vi "Generic command handler.vi"(8 "error in (no error)":errorcluster, 10 "Message in":refnum<class "GenericMessage.lvclass">, 11 "Tomo in":refnum<class "Tomo.lvclass">) -> (0 "error out":errorcluster, 2 "value":string, 3 "Tomo out":refnum<class "Tomo.lvclass">)   [LabVIEW 2012, in "Tomo.lvclass"]
doc: "The generic_command_handler processes the command 'generic'. Commands which are not part of the predefined list of commands fall under the 'generic' command for special activity."
uses:
  Tomo.lvclass
  <vilib>/Distrio/Murmex/GenericMessage/GenericMessage.lvclass
  <vilib>/Distrio/Murmex/Murmex/Murmex.lvclass
  Tomo.lvclass/Tomo.ctl
  <vilib>/Distrio/Murmex/StartMessage/StartMessage.lvclass
  Current activity.ctl
  file type.ctl
  notice type.ctl
  <vilib>/Distrio/Murmex/StopMessage/StopMessage.lvclass
  <vilib>/Distrio/Murmex/Message/Add or replace parameter.vi
  <vilib>/Distrio/Murmex/Message/Message.lvclass
  <vilib>/vision/NI_Vision_Development_Module.lvlib
panel:
  out "Image 2":T1(plugin-control)
  out "Image":T1(plugin-control)
  # "This method is called when the GENERIC\ntrigger is sent. \n\nOverride this method when your component needs to\nrespond to this trigger. \n\nCall parent for proper implementation"
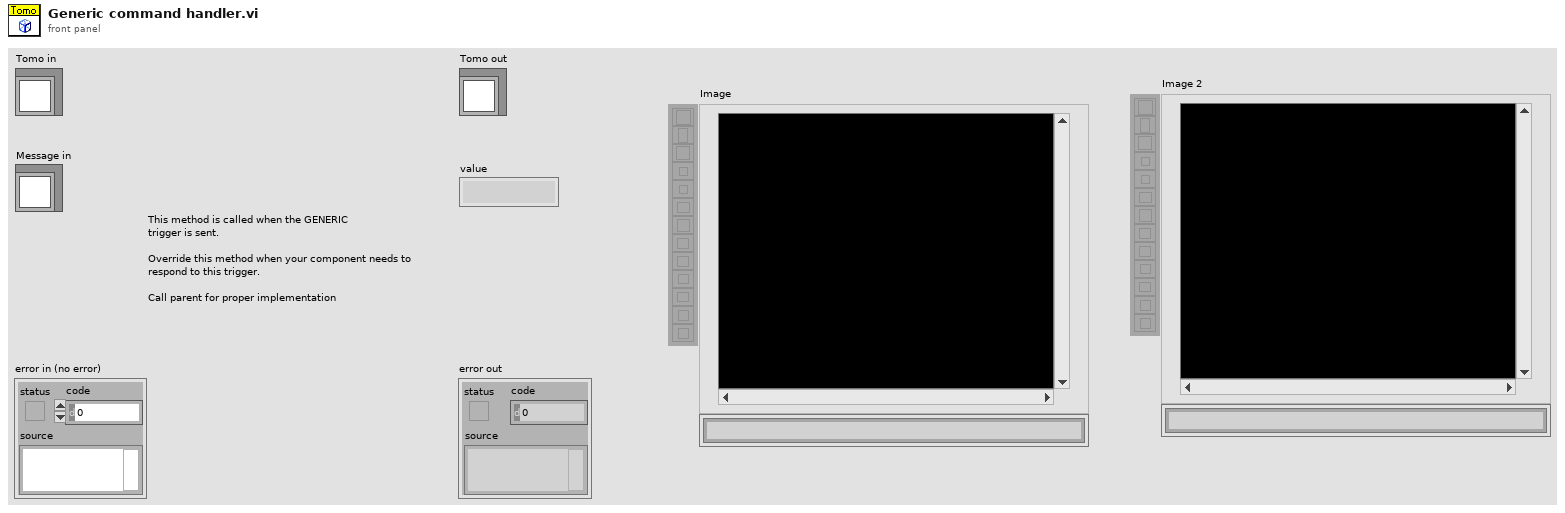
[diagram p1: front panel]
types:
  T1 = typedef "IMAQ Image.ctl" = refnum<image>
  T2 = typedef "Tomo.lvclass/Current activity.ctl" = enum16{"Idle", "Inter-stack motion", "Pre-tomo calculation", "Stack acquisition", "Stack preparation", "Pre-tomo stack acq", "Pre-tomo inter-stack"}
  T3 = typedef "Tomo.lvclass/file type.ctl" = enum16{"Volume map", "Completed stacks"}
  T4 = typedef "Tomo.lvclass/notice type.ctl" = enum16{"Tomography stopped", "Tomography error", "Tomography finished", "Timing issue", "Critical timing issue"}
  T5 = typedef "Tomo.lvclass/volume map.ctl" = enum16{"Cubic volume", "Custom volume", "Self-generate volume", "Time- tomography"}
  T6 = cluster{"Mean Value":sgl, "Standard Variation":sgl, "Minimal Value":sgl, "Maximal Value":sgl, "Area (calibrated)":sgl, "Area (pixels)":u32, "%":sgl, "Calibration Valid":bool}
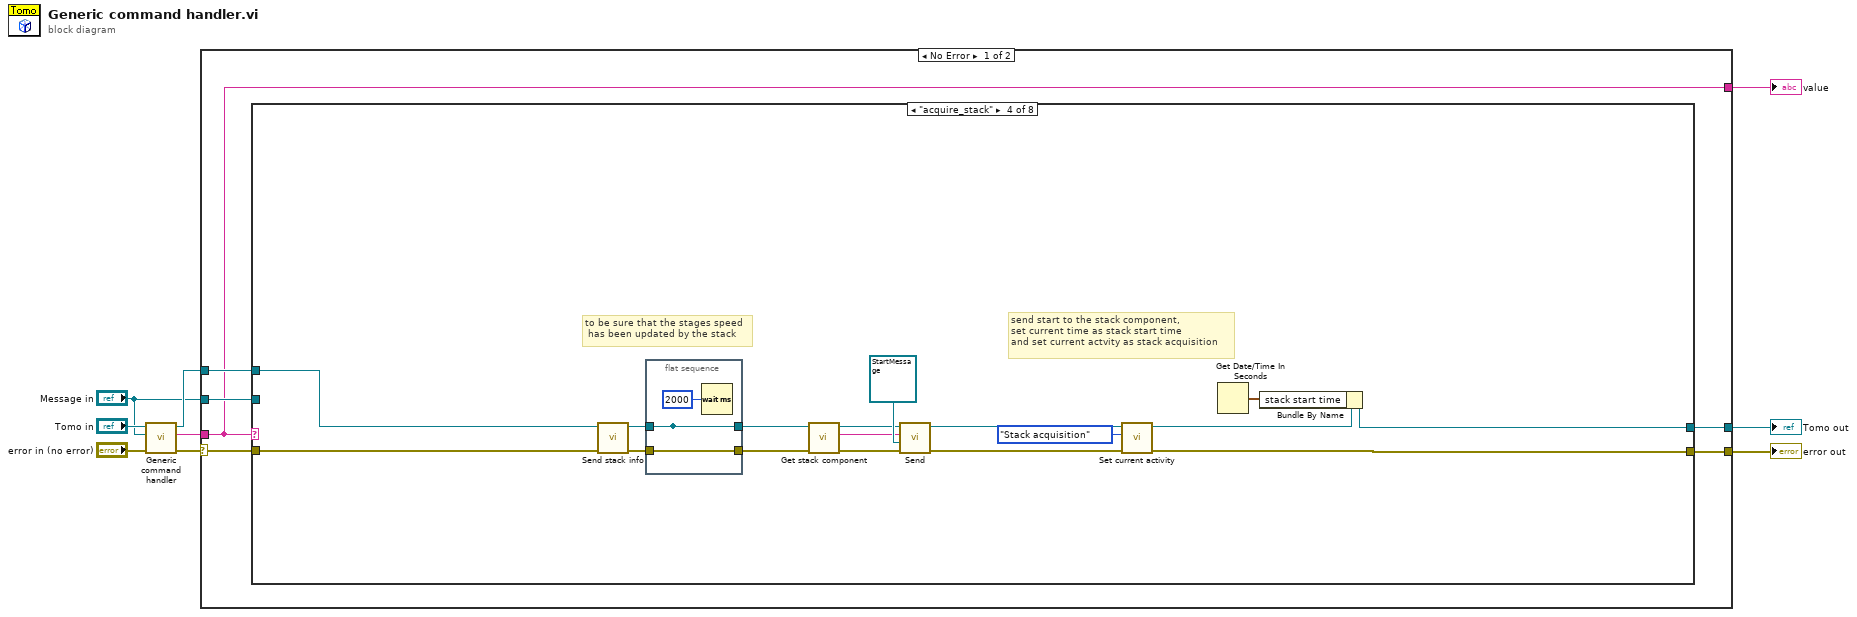
[diagram p0: block diagram]
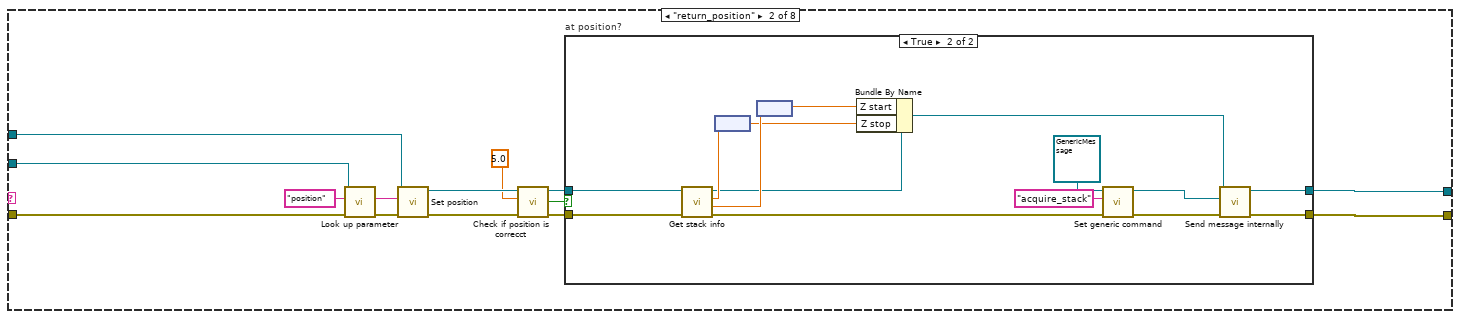
[diagram p3: hidden frame]
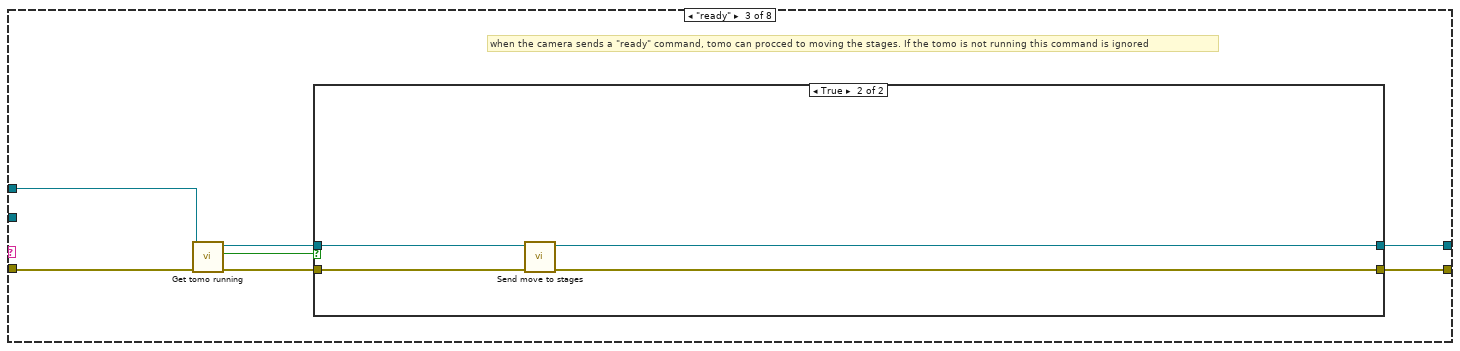
[diagram p5: hidden frame]
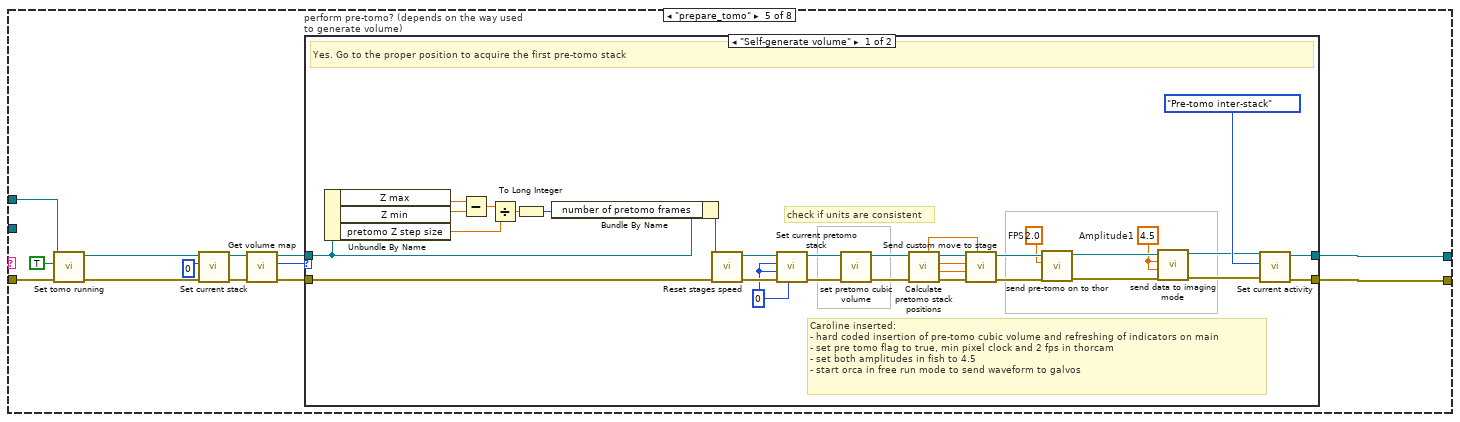
[diagram p7: hidden frame]
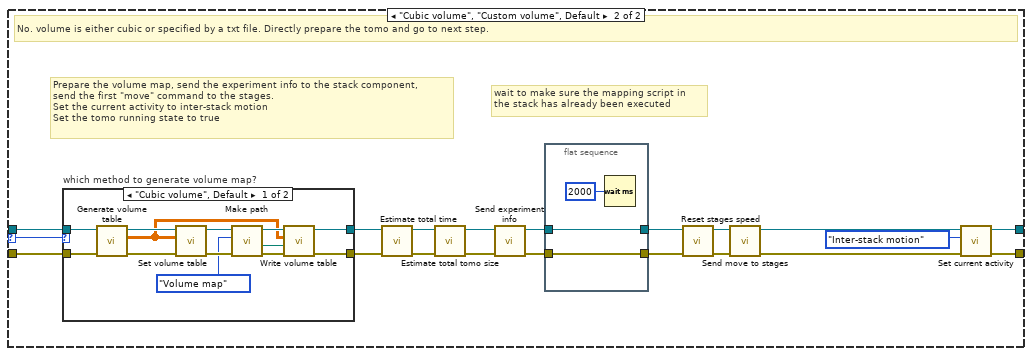
[diagram p8: hidden frame]
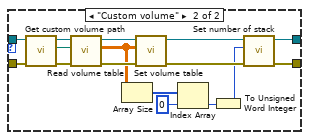
[diagram p9: hidden frame]
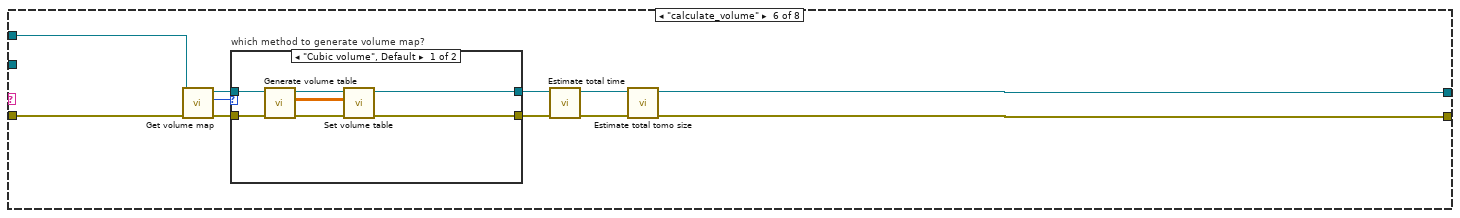
[diagram p10: hidden frame]
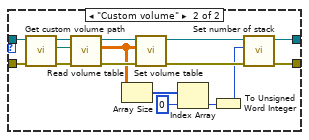
[diagram p11: hidden frame]
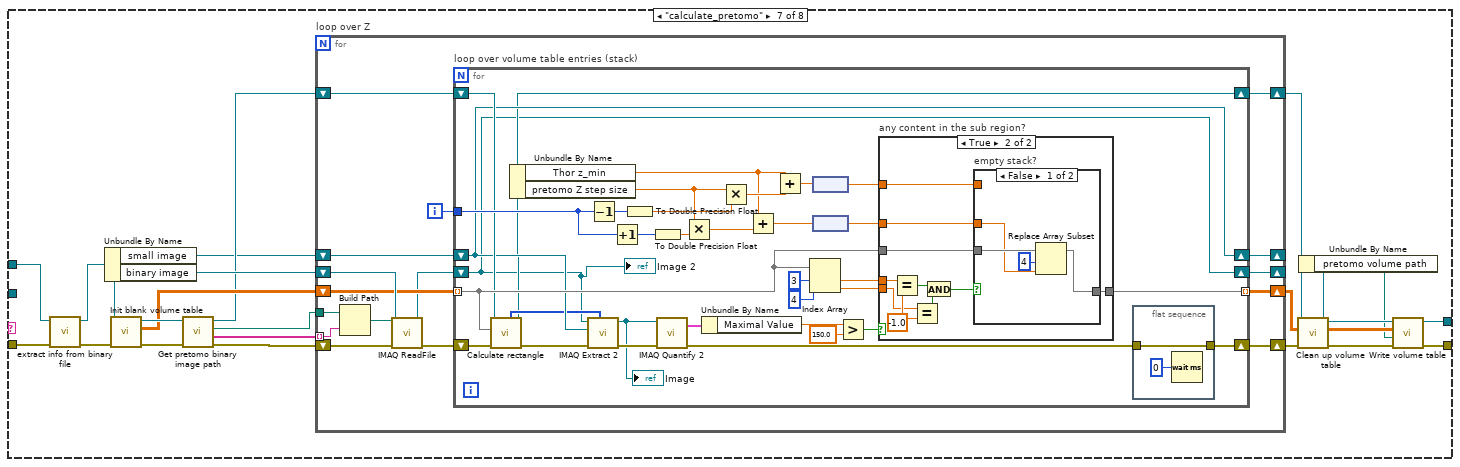
[diagram p12: hidden frame]
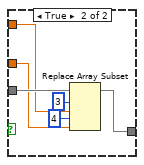
[diagram p14: hidden frame]
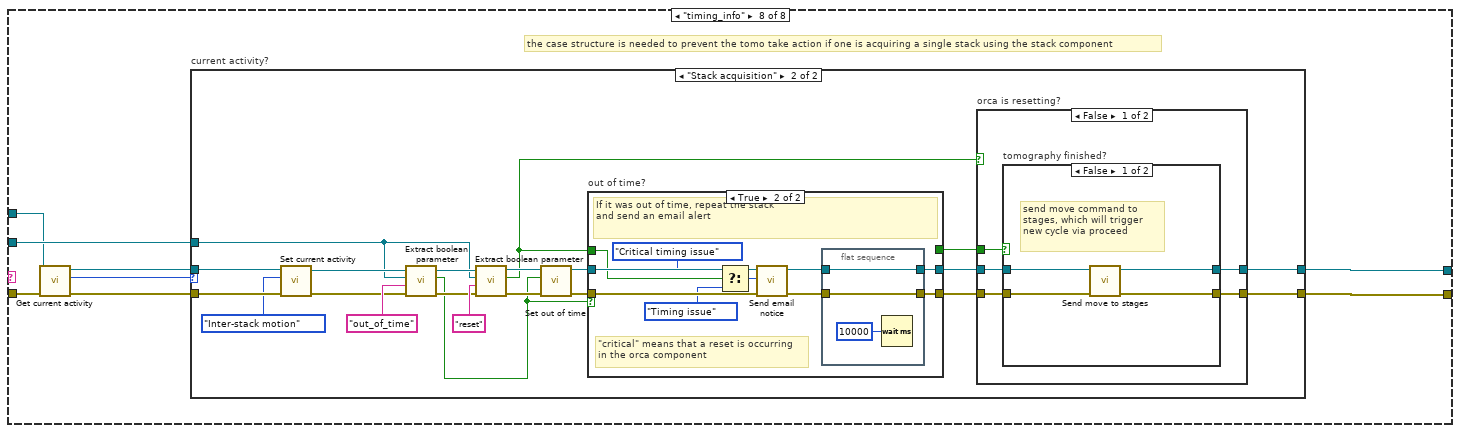
[diagram p15: hidden frame]
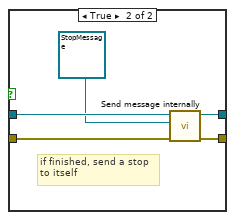
[diagram p17: hidden frame]
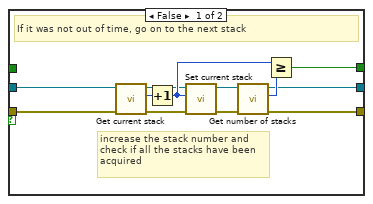
[diagram p19: hidden frame]
diagram:
  n1 = call-parent "Generic command handler.vi"("error in (no error)"="error in (no error)", "Message in"="Message in", "Murmex in"="Tomo in") -> ("error out"=w7:errorcluster, "value"=w6:string, "Murmex out"=w5:refnum<class "Tomo.lvclass">)  [unwired: 6 in]
  n2 = case shown="No Error" w7 {
    selector: w7 -> [w15 w380]
    tunnel: w6 -> [w11 w382]
    tunnel: w5 -> [w14 w381]
    tunnel: "Message in" -> [w13 _]
    tunnel: [w12 w381] -> w3
    tunnel: [w11 w382] -> w2
    tunnel: [w10 w380] -> w1
    frame No Error {
      n3 = case shown="\"acquire_stack\"" w11 {
        tunnel: w15 -> [w17 w31 w55 w62 w85 w182 w219 w312]
        tunnel: w14 -> [w16 w30 w54 w63 w86 w181 w217 w310]
        tunnel: w13 -> [_ w29 _ _ _ _ _ w315]
        tunnel: [w17 w19 w51 w75 w84 w179 w223 w313] -> w10
        tunnel: [w16 w18 w49 w64 w83 w180 w225 w314] -> w12
        frame Default {
        }
        frame "return_position" {
          n4 = call <vilib>:"Look up parameter.vi"("error in (no error)"=w31, "name"="position", "Message in"=w29) -> ("error out"=w27:errorcluster, "key"=w26:string)  [unwired: 5 in, 2 out]
          n5 = call-dynamic "Set position.vi"("error in (no error)"=w27, "XML in"=w26, "Tomo in"=w30) -> ("error out"=w25:errorcluster, "Tomo out"=w24:refnum<class "Tomo.lvclass">)  [unwired: 7 in]
          n6 = call-dynamic "Check if position is correcct.vi"("error in (no error)"=w25, "Tolerance (um)"=5.0 ("Tolerance"), "Tomo in"=w24) -> ("error out"=w21:errorcluster, "correct?"=w22:bool, "Tomo out"=w20:refnum<class "Tomo.lvclass">)  [unwired: 6 in]
          n7 = case "at position?" shown="True" w22 {
            tunnel: w21 -> [w33 w34]
            tunnel: w20 -> [w32 w35]
            tunnel: [w33 w48] -> w19
            tunnel: [w32 w47] -> w18
            frame False {
            }
            frame True {
              n8 = call-dynamic "Get stack info.vi"("error in (no error)"=w34, "Tomo in"=w35) -> ("error out"=w38:errorcluster, "Z start"=w45:dbl, "Z stop"=w46:dbl, "Tomo out"=w36:refnum<class "Tomo.lvclass">)  [unwired: 4 in, 2 out]
              n9 = node(w46) -> (w43:dbl[unit])
              n10 = node(w45) -> (w44:dbl[unit])
              n11 = Bundle By Name(cluster=w36, "Z start"=w44, "Z stop"=w43) -> (w37:refnum<class "Tomo.lvclass">)
              n12 = call <vilib>:"Set generic command.vi"("error in (no error)"=w38, "generic command"="acquire_stack", "GenericMessage in"=refnum<class "GenericMessage.lvclass"> refnum ("Distrio Murmex 1.2:GenericMessage")) -> ("error out"=w42:errorcluster, "GenericMessage out"=w39:refnum<class "GenericMessage.lvclass">)  [unwired: 7 in]
              n13 = call <vilib>:"Send message internally.vi"("error in (no error)"=w42, "Message"=w39, "Murmex in"=w37) -> ("error out"=w48:errorcluster, "Murmex out"=w47:refnum<class "Tomo.lvclass">)  [unwired: 7 in]
            }
          }
        }
        frame "ready" {
          # "when the camera sends a \"ready\" command, tomo can procced to moving the stages. If the tomo is not running this command is ignored"
          n14 = call-dynamic "Get tomo running.vi"("error in (no error)"=w55, "Tomo in"=w54) -> ("error out"=w52:errorcluster, "tomo running?"=w53:bool, "Tomo out"=w50:refnum<class "Tomo.lvclass">)  [unwired: 7 in]
          n15 = case shown="True" w53 {
            tunnel: w52 -> [w56 w61]
            tunnel: [w56 w60] -> w51
            tunnel: w50 -> [w57 w59]
            tunnel: [w57 w58] -> w49
            frame False {
            }
            frame True {
              n16 = call-dynamic "Send move to stages.vi"("error in (no error)"=w61, "Tomo in"=w59) -> ("error out"=w60:errorcluster, "Tomo out"=w58:refnum<class "Tomo.lvclass">)  [unwired: 8 in]
            }
          }
        }
        frame "acquire_stack" {
          # "to be sure that the stages speed\n has been updated by the stack"
          # "send start to the stack component,\nset current time as stack start time\nand set current actvity as stack acquisition"
          n17 = call-dynamic "Send stack info.vi"("error in (no error)"=w62, "Tomo in"=w63) -> ("error out"=w70:errorcluster, "Tomo out"=w69:refnum<class "Tomo.lvclass">)  [unwired: 8 in]
          n18 = flat-sequence {
            tunnel: [w81] -> w66
            tunnel: w70 -> [w81]
            tunnel: w69 -> [w79]
            tunnel: [w79] -> _
            tunnel: [w79] -> w67
            frame #0 {
              n19 = Wait (ms)(milliseconds to wait=u32 2000) -> ()  [unwired: 1 out]
            }
          }
          n20 = call-dynamic "Get stack component.vi"("error in (no error)"=w66, "Tomo in"=w67) -> ("error out"=w71:errorcluster, "stack component"=w77:string, "Tomo out"=w72:refnum<class "Tomo.lvclass">)  [unwired: 7 in]
          n21 = call <vilib>:"Send.vi"("error in (no error)"=w71, "Message"=refnum<class "StartMessage.lvclass"> refnum ("Message in"), "recipient"=w77, "Murmex in"=w72) -> ("error out"=w76:errorcluster, "Murmex out"=w74:refnum<class "Tomo.lvclass">)  [unwired: 6 in]
          n22 = call-dynamic "Set current activity.vi"("error in (no error)"=w76, "Current activity"=Current_activity."Stack acquisition", "Tomo in"=w74) -> ("error out"=w75:errorcluster, "Tomo out"=w65:refnum<class "Tomo.lvclass">)  [unwired: 7 in]
          n23 = Get Date/Time In Seconds() -> (seconds since 1Jan1904=w68:timestamp)
          n24 = Bundle By Name(cluster=w65, "stack start time"=w68) -> (w64:refnum<class "Tomo.lvclass">)
        }
        frame "prepare_tomo" {
          n25 = call-dynamic "Set tomo running.vi"("error in (no error)"=w85, "tomo running?"=TRUE, "Tomo in"=w86) -> ("error out"=w87:errorcluster, "Tomo out"=w88:refnum<class "Tomo.lvclass">)  [unwired: 7 in]
          n26 = call-dynamic "Set current stack.vi"("error in (no error)"=w87, "Current stack"=u16 0, "Tomo in"=w88) -> ("error out"=w91:errorcluster, "Tomo out"=w92:refnum<class "Tomo.lvclass">)  [unwired: 7 in]
          n27 = call-dynamic "Get volume map.vi"("error in (no error)"=w91, "Tomo in"=w92) -> ("error out"=w94:errorcluster, "Volume map"=w82:T5, "Tomo out"=w93:refnum<class "Tomo.lvclass">)  [unwired: 7 in]
          n28 = case "perform pre-tomo? (depends on the way used to generate volume)" shown="\"Self-generate volume\"" w82 {
            selector: w82 -> [_ w127]
            tunnel: w94 -> [w107 w146]
            tunnel: w93 -> [w108 w145]
            tunnel: [w119 w137] -> w84
            tunnel: [w118 w135] -> w83
            frame "Self-generate volume" {
              w101 = 2.0  # FPS
              w102 = 4.5  # Amplitude1
              w109 = 0 ("current x stack")
              # "Caroline inserted:\n- hard coded insertion of pre-tomo cubic volume and refreshing of indicators on main\n- set pre tomo flag to true, min pixel clock and 2 fps in thorcam\n- set both amplitudes in fish to 4.5\n- start orca in free run mode to send waveform to galvos"
              # "check if units are consistent"
              # "Yes. Go to the proper position to acquire the first pre-tomo stack"
              n29 = Unbundle By Name(w108) -> ("Z max"=w116:dbl[unit], "Z min"=w115:dbl[unit], "pretomo Z step size"=w113:dbl[unit])
              n30 = Subtract(x=w116, y=w115) -> (x-y=w114:dbl[unit])
              n31 = Divide(x=w114, y=w113) -> (x/y=w110:dbl)
              n32 = To Long Integer(number=w110) -> (32bit integer=w111:i32)
              n33 = Bundle By Name(cluster=w108, "number of pretomo frames"=w111) -> (w112:refnum<class "Tomo.lvclass">)
              n34 = call-dynamic "Reset stages speed.vi"("error in (no error)"=w107, "Tomo in"=w112) -> ("error out"=w126:errorcluster, "Tomo out"=w125:refnum<class "Tomo.lvclass">)  [unwired: 8 in]
              n35 = call-dynamic "Set current pretomo stack.vi"("z step number"=w109, "error in (no error)"=w126, "current y stack"=w109, "current x stack"=w109, "Tomo in"=w125) -> ("error out"=w98:errorcluster, "Tomo out"=w100:refnum<class "Tomo.lvclass">)  [unwired: 5 in]
              n36 = call-dynamic "set pretomo cubic volume.vi"("error in (no error)"=w98, "Tomo in"=w100) -> ("error out"=w97:errorcluster, "Tomo out"=w99:refnum<class "Tomo.lvclass">)  [unwired: 8 in]
              n37 = call-dynamic "Calculate pretomo stack positions.vi"("error in (no error)"=w97, "Tomo in"=w99) -> ("error out"=w123:errorcluster, "Y pos"=w120:dbl[unit], "X pos"=w121:dbl[unit], "Tomo out"=w124:refnum<class "Tomo.lvclass">, "Z pos"=w122:dbl[unit])  [unwired: 5 in]
              n38 = call-dynamic "Send custom move to stage.vi"("Z pos"=w122, "error in (no error)"=w123, "Y pos"=w120, "X pos"=w121, "Tomo in"=w124) -> ("error out"=w106:errorcluster, "Tomo out"=w105:refnum<class "Tomo.lvclass">)  [unwired: 5 in]
              n39 = call-dynamic "send pre-tomo on to thor.vi"("error in (no error)"=w106, "FPS"=w101, "Tomo in"=w105) -> ("error out"=w103:errorcluster, "Tomo out"=w104:refnum<class "Tomo.lvclass">)  [unwired: 7 in]
              n40 = call-dynamic "send data to imaging mode.vi"("error in (no error)"=w103, "Amplitude2"=w102, "Amplitude1"=w102, "Tomo in"=w104) -> ("error out"=w96:errorcluster, "Tomo out"=w95:refnum<class "Tomo.lvclass">)  [unwired: 6 in]
              n41 = call-dynamic "Set current activity.vi"("error in (no error)"=w96, "Current activity"=Current_activity."Pre-tomo inter-stack", "Tomo in"=w95) -> ("error out"=w119:errorcluster, "Tomo out"=w118:refnum<class "Tomo.lvclass">)  [unwired: 7 in]
            }
            frame "Cubic volume", "Custom volume", Default {
              # "wait to make sure the mapping script in \nthe stack has already been executed"
              # "Prepare the volume map, send the experiment info to the stack component,\nsend the first \"move\" command to the stages.\nSet the current activity to inter-stack motion\nSet the tomo running state to true"
              # "No. volume is either cubic or specified by a txt file. Directly prepare the tomo and go to next step."
              n42 = case "which method to generate volume map?" shown="\"Cubic volume\", Default" w127 {
                tunnel: w146 -> [w161 w176]
                tunnel: w145 -> [w162 w174]
                tunnel: [w151 w168] -> w143
                tunnel: [w150 w170] -> w144
                frame "Cubic volume", Default {
                  n43 = call-dynamic "Generate volume table.vi"("error in (no error)"=w161, "Tomo in"=w162) -> ("error out"=w159:errorcluster, "Volume table"=w152:dbl[][], "Tomo out"=w160:refnum<class "Tomo.lvclass">)  [unwired: 7 in]
                  n44 = call-dynamic "Set volume table.vi"("error in (no error)"=w159, "Volume map in"=w152, "Tomo in"=w160) -> ("error out"=w157:errorcluster, "Tomo out"=w158:refnum<class "Tomo.lvclass">)  [unwired: 7 in]
                  n45 = call-dynamic "Make path.vi"("error in (no error)"=w157, "File type"=file_type."Volume map", "Tomo in"=w158) -> ("error out"=w154:errorcluster, "path"=w153:path, "Tomo out"=w155:refnum<class "Tomo.lvclass">)  [unwired: 6 in]
                  n46 = call-dynamic "Write volume table.vi"("error in (no error)"=w154, "File name"=w153, "Volume map"=w152, "Tomo in"=w155) -> ("error out"=w150:errorcluster, "Tomo out"=w151:refnum<class "Tomo.lvclass">)  [unwired: 6 in]
                }
                frame "Custom volume" {
                  n47 = call-dynamic "Get custom volume path.vi"("error in (no error)"=w176, "Tomo in"=w174) -> ("error out"=w175:errorcluster, "Custom volume path"=w172:path, "Tomo out"=w173:refnum<class "Tomo.lvclass">)  [unwired: 7 in]
                  n48 = call "Read volume table.vi"("error in (no error)"=w175, "File path"=w172, "Tomo in"=w173) -> ("error out"=w177:errorcluster, "System Array"=w164:dbl[][], "Tomo out"=w178:refnum<class "Tomo.lvclass">)  [unwired: 6 in]
                  n49 = Array Size(array=w164) -> (size(s)=w167:i32[])
                  n50 = call-dynamic "Set volume table.vi"("error in (no error)"=w177, "Volume map in"=w164, "Tomo in"=w178) -> ("error out"=w171:errorcluster, "Tomo out"=w169:refnum<class "Tomo.lvclass">)  [unwired: 7 in]
                  n51 = Index Array(array=w167, index=0) -> (element=w165:i32)
                  n52 = To Unsigned Word Integer(number=w165) -> (unsigned 16bit integer=w163:u16)
                  n53 = call-dynamic "Set number of stack.vi"("error in (no error)"=w171, "Number of stacks"=w163, "Tomo in"=w169) -> ("error out"=w170:errorcluster, "Tomo out"=w168:refnum<class "Tomo.lvclass">)  [unwired: 7 in]
                }
              }
              n54 = call-dynamic "Estimate total time.vi"("error in (no error)"=w144, "Tomo in"=w143) -> ("error out"=w131:errorcluster, "Tomo out"=w133:refnum<class "Tomo.lvclass">)  [unwired: 7 in, 1 out]
              n55 = call "Estimate total tomo size.vi"("error in (no error)"=w131, "Tomo in"=w133) -> ("error out"=w130:errorcluster, "Tomo out"=w132:refnum<class "Tomo.lvclass">)  [unwired: 7 in, 1 out]
              n56 = call-dynamic "Send experiment info.vi"("error in (no error)"=w130, "Tomo in"=w132) -> ("error out"=w138:errorcluster, "Tomo out"=w140:refnum<class "Tomo.lvclass">)  [unwired: 8 in]
              n57 = flat-sequence {
                tunnel: [w149] -> w141
                tunnel: w140 -> [w149]
                tunnel: [w148] -> w139
                tunnel: w138 -> [w148]
                frame #0 {
                  n58 = Wait (ms)(milliseconds to wait=u32 2000) -> ()  [unwired: 1 out]
                }
              }
              n59 = call-dynamic "Reset stages speed.vi"("error in (no error)"=w139, "Tomo in"=w141) -> ("error out"=w129:errorcluster, "Tomo out"=w128:refnum<class "Tomo.lvclass">)  [unwired: 8 in]
              n60 = call-dynamic "Send move to stages.vi"("error in (no error)"=w129, "Tomo in"=w128) -> ("error out"=w142:errorcluster, "Tomo out"=w136:refnum<class "Tomo.lvclass">)  [unwired: 8 in]
              n61 = call-dynamic "Set current activity.vi"("error in (no error)"=w142, "Current activity"=Current_activity."Inter-stack motion", "Tomo in"=w136) -> ("error out"=w137:errorcluster, "Tomo out"=w135:refnum<class "Tomo.lvclass">)  [unwired: 7 in]
            }
          }
        }
        frame "calculate_volume" {
          n62 = call-dynamic "Get volume map.vi"("error in (no error)"=w182, "Tomo in"=w181) -> ("error out"=w188:errorcluster, "Volume map"=w189:T5, "Tomo out"=w187:refnum<class "Tomo.lvclass">)  [unwired: 7 in]
          n63 = case "which method to generate volume map?" shown="\"Cubic volume\", Default" w189 {
            tunnel: w188 -> [w195 w210]
            tunnel: w187 -> [w196 w208]
            tunnel: [w191 w202] -> w185
            tunnel: [w190 w204] -> w186
            frame "Cubic volume", Default {
              n64 = call-dynamic "Generate volume table.vi"("error in (no error)"=w195, "Tomo in"=w196) -> ("error out"=w193:errorcluster, "Volume table"=w192:dbl[][], "Tomo out"=w194:refnum<class "Tomo.lvclass">)  [unwired: 7 in]
              n65 = call-dynamic "Set volume table.vi"("error in (no error)"=w193, "Volume map in"=w192, "Tomo in"=w194) -> ("error out"=w190:errorcluster, "Tomo out"=w191:refnum<class "Tomo.lvclass">)  [unwired: 7 in]
            }
            frame "Custom volume" {
              n66 = call-dynamic "Get custom volume path.vi"("error in (no error)"=w210, "Tomo in"=w208) -> ("error out"=w209:errorcluster, "Custom volume path"=w206:path, "Tomo out"=w207:refnum<class "Tomo.lvclass">)  [unwired: 7 in]
              n67 = call "Read volume table.vi"("error in (no error)"=w209, "File path"=w206, "Tomo in"=w207) -> ("error out"=w211:errorcluster, "System Array"=w198:dbl[][], "Tomo out"=w212:refnum<class "Tomo.lvclass">)  [unwired: 6 in]
              n68 = Array Size(array=w198) -> (size(s)=w201:i32[])
              n69 = call-dynamic "Set volume table.vi"("error in (no error)"=w211, "Volume map in"=w198, "Tomo in"=w212) -> ("error out"=w205:errorcluster, "Tomo out"=w203:refnum<class "Tomo.lvclass">)  [unwired: 7 in]
              n70 = Index Array(array=w201, index=0) -> (element=w199:i32)
              n71 = To Unsigned Word Integer(number=w199) -> (unsigned 16bit integer=w197:u16)
              n72 = call-dynamic "Set number of stack.vi"("error in (no error)"=w205, "Number of stacks"=w197, "Tomo in"=w203) -> ("error out"=w204:errorcluster, "Tomo out"=w202:refnum<class "Tomo.lvclass">)  [unwired: 7 in]
            }
          }
          n73 = call-dynamic "Estimate total time.vi"("error in (no error)"=w186, "Tomo in"=w185) -> ("error out"=w183:errorcluster, "Tomo out"=w184:refnum<class "Tomo.lvclass">)  [unwired: 7 in, 1 out]
          n74 = call "Estimate total tomo size.vi"("error in (no error)"=w183, "Tomo in"=w184) -> ("error out"=w179:errorcluster, "Tomo out"=w180:refnum<class "Tomo.lvclass">)  [unwired: 7 in, 1 out]
        }
        frame "calculate_pretomo" {
          n75 = call-dynamic "extract info from binary file.vi"("error in (no error)"=w219, "Tomo in"=w217) -> ("error out"=w218:errorcluster, "Tomo out"=w216:refnum<class "Tomo.lvclass">)  [unwired: 8 in]
          n76 = Unbundle By Name(w216) -> ("small image"=w229:T1, "binary image"=w232:T1)
          n77 = call-dynamic "Init blank volume table.vi"("error in (no error)"=w218, "Tomo in"=w216) -> ("error out"=w233:errorcluster, "blank volume table"=w231:dbl[][], "Tomo out"=w234:refnum<class "Tomo.lvclass">)  [unwired: 7 in]
          n78 = call-dynamic "Get pretomo binary image path.vi"("error in (no error)"=w233, "Tomo in"=w234) -> ("error out"=w215:errorcluster, "filenames"=w214:string[], "pretomo binary path"=w213:path, "Tomo out"=w230:refnum<class "Tomo.lvclass">)  [unwired: 6 in]
          n79 = for "loop over Z" {
            shift-right: [w239] -> w227
            shift-left: w215 -> [w250]
            shift-right: [w241] -> w226
            shift-left: w231 -> [w247]
            shift-right: [w240] -> w228
            shift-left: w230 -> [w245]
            shift-right: [w238] -> _
            shift-left: w229 -> [w243]
            shift-right: [w237] -> _
            shift-left: w232 -> [w249]
            tunnel: w214 -> [w236] mode=indexing
            tunnel: w213 -> [w235]
            i -> [w242]
            n80 = Build Path(base path=w235, name or relative path=w236) -> (appended path=w248:path)
            n81 = call "IMAQ ReadFile"("File Path"=w248, "error in (no error)"=w250, "Image"=w249) -> ("error out"=w246:errorcluster, "Image Out"=w244:T1)  [unwired: 4 in, 3 out]
            n82 = for "loop over volume table entries (stack)" {
              tunnel: w247 -> [w273] mode=indexing
              shift-right: [w254] -> w239
              shift-left: w246 -> [w284]
              tunnel: w242 -> [w268]
              tunnel: [w259] -> w241 mode=indexing
              shift-right: [w255] -> w240
              shift-left: w245 -> [w258]
              shift-right: [w257] -> w238
              shift-left: w243 -> [w257]
              shift-right: [w251] -> w237
              shift-left: w244 -> [w251]
              n83 = call-dynamic "Calculate rectangle.vi"("error in (no error)"=w284, "xyzs array"=w273, "Tomo in"=w258) -> ("error out"=w283:errorcluster, "Tomo out"=w255:refnum<class "Tomo.lvclass">, "rectangle"=w256:i32[])  [unwired: 6 in]
              n84 = Unbundle By Name(w255) -> ("Thor z_min"=w261:dbl[unit], "pretomo Z step size"=w265:dbl[unit])
              n85 = call "IMAQ Extract 2"("Optional Rectangle"=w256, "error in (no error)"=w283, "Image Dst"=w257, "Image Src"=w251) -> ("error out"=w282:errorcluster, "Image Dst Out"=w252:T1)  [unwired: 6 in]
              "Image" <- w252
              n86 = Decrement(x=w268) -> (x-1=w271:i32)
              n87 = Increment(x=w268) -> (x+1=w267:i32)
              n88 = To Double Precision Float(number=w271) -> (double precision float=w272:dbl)
              n89 = To Double Precision Float(number=w267) -> (double precision float=w266:dbl)
              n90 = call "IMAQ Quantify 2"("error in (no error)"=w282, "Image"=w252) -> ("error out"=w253:errorcluster, "Global Report"=w281:T6)  [unwired: 7 in, 1 out]
              n91 = Multiply(x=w265, y=w266) -> (x*y=w263:dbl[unit])
              n92 = Unbundle By Name(w281) -> ("Maximal Value"=w278:sgl)
              n93 = Multiply(x=w265, y=w272) -> (x*y=w264:dbl[unit])
              n94 = Add(x=w261, y=w263) -> (x+y=w262:dbl[unit])
              n95 = Add(x=w261, y=w264) -> (x+y=w270:dbl[unit])
              n96 = Index Array(array=w273, index #1=3 ("index"), index #2=4 ("index")) -> (element #1=w275:dbl, element #2=w274:dbl)
              n97 = node(w270) -> (w269:dbl)
              n98 = node(w262) -> (w260:dbl)
              n99 = Greater?(x=w278, y=sgl 150.0) -> (0:w276:bool)
              n100 = case "any content in the sub region?" shown="True" w276 {
                tunnel: w275 -> [_ w297]
                tunnel: w274 -> [_ w295]
                tunnel: w273 -> [w287 w294]
                tunnel: w269 -> [_ w293]
                tunnel: w260 -> [_ w291]
                tunnel: [w287 w292] -> w259
                frame False {
                }
                frame True {
                  w296 = -1.0 ("y")
                  n101 = Equal?(x=w297, y=w296) -> (x = y?=w289:bool)
                  n102 = Equal?(x=w295, y=w296) -> (x = y?=w290:bool)
                  n103 = And(x=w289, y=w290) -> (x .and. y?=w288:bool)
                  n104 = case "empty stack?" shown="False" w288 {
                    tunnel: w294 -> [w300 w307]
                    tunnel: w293 -> [_ w305]
                    tunnel: [w298 w304] -> w292
                    tunnel: w291 -> [w299 w302]
                    frame False {
                      n105 = Replace Array Subset(array=w300, new element=w299, index=4) -> (w298:dbl[])
                    }
                    frame True {
                      n106 = Replace Array Subset(array=w307, new element #1=w305, index #1=3 ("index"), new element #2=w302, index #2=4 ("index")) -> (w304:dbl[])
                    }
                  }
                }
              }
              n107 = flat-sequence {
                tunnel: [w286] -> w254
                tunnel: w253 -> [w286]
                frame #0 {
                  n108 = Wait (ms)(milliseconds to wait=u32 0) -> ()  [unwired: 1 out]
                }
              }
              "Image 2" <- w251
            }
          }
          n109 = call-dynamic "Clean up volume table.vi"("error in (no error)"=w227, "Volume table in"=w226, "Tomo in"=w228) -> ("error out"=w224:errorcluster, "Volume table out"=w222:dbl[][], "Tomo out"=w221:refnum<class "Tomo.lvclass">)  [unwired: 6 in]
          n110 = Unbundle By Name(w221) -> ("pretomo volume path"=w220:path)
          n111 = call-dynamic "Write volume table.vi"("error in (no error)"=w224, "File name"=w220, "Volume map"=w222, "Tomo in"=w221) -> ("error out"=w223:errorcluster, "Tomo out"=w225:refnum<class "Tomo.lvclass">)  [unwired: 6 in]
        }
        frame "timing_info" {
          # "the case structure is needed to prevent the tomo take action if one is acquiring a single stack using the stack component"
          n112 = call-dynamic "Get current activity.vi"("error in (no error)"=w312, "Tomo in"=w310) -> ("error out"=w311:errorcluster, "Current activity"=w308:T2, "Tomo out"=w309:refnum<class "Tomo.lvclass">)  [unwired: 7 in]
          n113 = case "current activity?" shown="\"Stack acquisition\"" w308 {
            tunnel: w315 -> [_ w320]
            tunnel: [w317 w336] -> w314
            tunnel: [w316 w335] -> w313
            tunnel: w311 -> [w316 w331]
            tunnel: w309 -> [w317 w330]
            frame "Idle", Default {
            }
            frame "Stack acquisition" {
              n114 = call-dynamic "Set current activity.vi"("error in (no error)"=w331, "Current activity"=Current_activity."Inter-stack motion", "Tomo in"=w330) -> ("error out"=w318:errorcluster, "Tomo out"=w322:refnum<class "Tomo.lvclass">)  [unwired: 7 in]
              n115 = call-dynamic "Extract boolean parameter.vi"("error in (no error)"=w318, "parameter"="out_of_time" ("name"), "Message in"=w320, "Tomo in"=w322) -> ("error out"=w324:errorcluster, "parameter"=w323:bool, "Tomo out"=w321:refnum<class "Tomo.lvclass">)  [unwired: 5 in]
              n116 = call-dynamic "Extract boolean parameter.vi"("error in (no error)"=w324, "parameter"="reset" ("name"), "Message in"=w320, "Tomo in"=w321) -> ("error out"=w328:errorcluster, "parameter"=w326:bool, "Tomo out"=w327:refnum<class "Tomo.lvclass">)  [unwired: 5 in]
              n117 = call-dynamic "Set out of time.vi"("error in (no error)"=w328, "out of time?"=w323, "Tomo in"=w327) -> ("error out"=w333:errorcluster, "Tomo out"=w332:refnum<class "Tomo.lvclass">)  [unwired: 7 in]
              n118 = case "out of time?" shown="True" w323 {
                tunnel: w333 -> [w359 w375]
                tunnel: w332 -> [w358 w376]
                tunnel: [w357 w370] -> w338
                tunnel: [w356 w368] -> w337
                tunnel: [w355 _] -> w334
                tunnel: w326 -> [_ w372]
                frame False {
                  # "increase the stack number and\ncheck if all the stacks have been\nacquired"
                  # "If it was not out of time, go on to the next stack"
                  n119 = call-dynamic "Get current stack.vi"("error in (no error)"=w359, "Tomo in"=w358) -> ("error out"=w361:errorcluster, "Current stack"=w362:u16, "Tomo out"=w360:refnum<class "Tomo.lvclass">)  [unwired: 7 in]
                  n120 = Increment(x=w362) -> (x+1=w366:u16)
                  n121 = call-dynamic "Set current stack.vi"("error in (no error)"=w361, "Current stack"=w366, "Tomo in"=w360) -> ("error out"=w363:errorcluster, "Tomo out"=w364:refnum<class "Tomo.lvclass">)  [unwired: 7 in]
                  n122 = call-dynamic "Get number of stacks.vi"("error in (no error)"=w363, "Tomo in"=w364) -> ("error out"=w357:errorcluster, "Number of stacks"=w365:u16, "Tomo out"=w356:refnum<class "Tomo.lvclass">)  [unwired: 7 in]
                  n123 = Greater Or Equal?(x=w366, y=w365) -> (x >= y?=w355:bool)
                }
                frame True {
                  # "\"critical\" means that a reset is occurring\nin the orca component"
                  # "If it was out of time, repeat the stack\nand send an email alert"
                  n124 = Select(t=notice_type."Critical timing issue" ("Notice type"), s=w372, f=notice_type."Timing issue" ("Notice type")) -> (s? t:f=w371:T4)
                  n125 = call-dynamic "Send email notice.vi"("error in (no error)"=w375, "Notice type"=w371, "Tomo in"=w376) -> ("error out"=w369:errorcluster, "Tomo out"=w367:refnum<class "Tomo.lvclass">)  [unwired: 7 in]
                  n126 = flat-sequence {
                    tunnel: [w379] -> w370
                    tunnel: w369 -> [w379]
                    tunnel: [w378] -> w368
                    tunnel: w367 -> [w378]
                    frame #0 {
                      n127 = Wait (ms)(milliseconds to wait=u32 10000) -> ()  [unwired: 1 out]
                    }
                  }
                }
              }
              n128 = case "orca is resetting?" shown="False" w326 {
                tunnel: w338 -> [w343 w354]
                tunnel: w337 -> [w342 w353]
                tunnel: [w341 w353] -> w336
                tunnel: [w340 w354] -> w335
                tunnel: w334 -> [w339 _]
                frame False {
                  n129 = case "tomography finished?" shown="False" w339 {
                    tunnel: w343 -> [w347 w352]
                    tunnel: w342 -> [w346 w349]
                    tunnel: [w345 w350] -> w341
                    tunnel: [w344 w351] -> w340
                    frame False {
                      # "send move command to stages, which will trigger new cycle via proceed"
                      n130 = call-dynamic "Send move to stages.vi"("error in (no error)"=w347, "Tomo in"=w346) -> ("error out"=w344:errorcluster, "Tomo out"=w345:refnum<class "Tomo.lvclass">)  [unwired: 8 in]
                    }
                    frame True {
                      # "if finished, send a stop\nto itself"
                      n131 = call <vilib>:"Send message internally.vi"("error in (no error)"=w352, "Message"=refnum<class "StopMessage.lvclass"> refnum ("Message in"), "Murmex in"=w349) -> ("error out"=w351:errorcluster, "Murmex out"=w350:refnum<class "Tomo.lvclass">)  [unwired: 7 in]
                    }
                  }
                }
                frame True {
                  # "do nothing. Orca will tell\nyou when it's ready"
                }
              }
            }
          }
        }
      }
    }
    frame Error {
    }
  }
  "error out" <- w1
  "Tomo out" <- w3
  "value" <- w2
